vi "read_pressure.vi"(8 "error in (no error)":errorcluster, 10 "Transmitter":string="001", 11 "VISA resource name":refnum<visa-resource-name>) -> (0 "error out":errorcluster, 1 "pressure mbar numeric":dbl format="%_4e", 3 "VISA resource name 2":refnum<visa-resource-name>)   [LabVIEW 2010]
panel:
  out "concatenated string":string
  out "octal integer string":string
  out "sum":u8
  out "unsigned byte array":u8[](array[numeric])
  out "Numeric":u8
  out "read buffer":string
  out "return count":u32
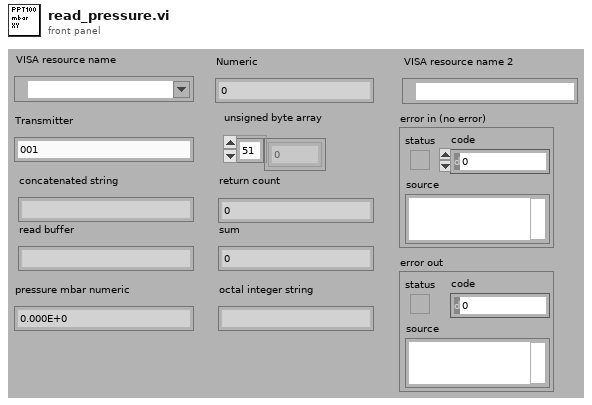
[diagram p1: front panel]
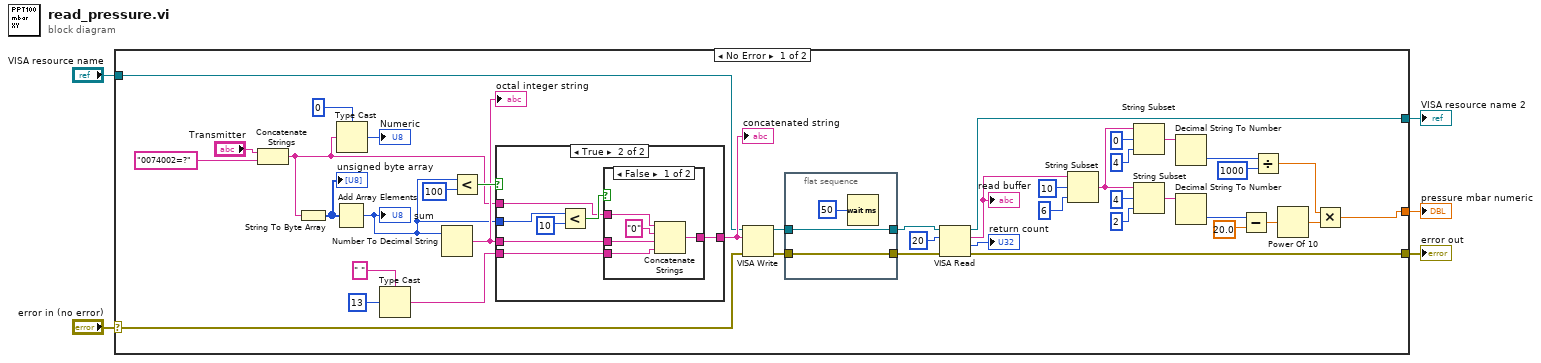
[diagram p0: block diagram]
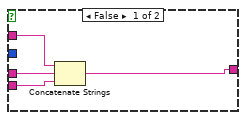
[diagram p2: hidden frame]
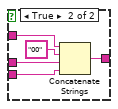
[diagram p3: hidden frame]
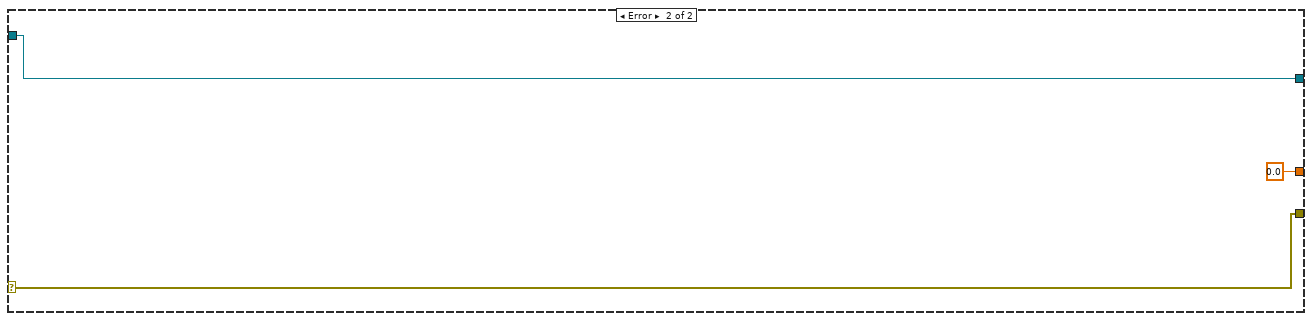
[diagram p4: hidden frame]
diagram:
  n1 = case shown="No Error" "error in (no error)" {
    selector: "error in (no error)" -> [w8 w73]
    tunnel: "VISA resource name" -> [w9 w74]
    tunnel: [w45 w73] -> w4
    tunnel: [w44 w74] -> w2
    tunnel: [w22 0.0] -> w1
    frame No Error {
      n2 = Concatenate Strings("Transmitter", "0074002=?") -> (w10:string)
      n3 = String To Byte Array(string=w10) -> (unsigned byte array=w17:u8[])
      "unsigned byte array" <- w17
      n4 = Add Array Elements(numeric array=w17) -> (sum=w12:u8)
      "sum" <- w12
      n5 = Type Cast(type=u8 0, x=w10) -> (*(type *) &x=→"Numeric":u8)
      n6 = Type Cast(type=" ", x=u8 13 ("Numeric 2")) -> (*(type *) &x=w14:string)
      n7 = Number To Decimal String(number=w12) -> (decimal integer string=w13:string)  [unwired: 1 in]
      "octal integer string" <- w13
      n8 = Less?(x=w12, y=u8 100) -> (x < y?=w15:bool)
      n9 = case shown="True" w15 {
        tunnel: w10 -> [w51 w53]
        tunnel: w14 -> [w49 w55]
        tunnel: w13 -> [w48 w54]
        tunnel: w12 -> [_ w58]
        tunnel: [w50 w52] -> w11
        frame False {
          n10 = Concatenate Strings(w51, w48, w49) -> (w50:string)
        }
        frame True {
          n11 = Less?(x=w58, y=u8 10) -> (x < y?=w56:bool)
          n12 = case shown="False" w56 {
            tunnel: w55 -> [w62 w67]
            tunnel: w54 -> [w61 w66]
            tunnel: w53 -> [w60 w65]
            tunnel: [w59 w64] -> w52
            frame False {
              n13 = Concatenate Strings(w60, "0" ("string"), w61, w62) -> (w59:string)
            }
            frame True {
              n14 = Concatenate Strings(w65, "00" ("string"), w66, w67) -> (w64:string)
            }
          }
        }
      }
      "concatenated string" <- w11
      n15 = VISA Write(VISA resource name=w9, write buffer=w11, error in (no error)=w8) -> (VISA resource name out=w7:refnum<visa-resource-name>, error out=w6:errorcluster)  [unwired: 1 out]
      n16 = flat-sequence {
        tunnel: [w69] -> w41
        tunnel: w6 -> [w70]
        tunnel: [w70] -> w42
        tunnel: w7 -> [w69]
        frame #0 {
          n17 = Wait (ms)(milliseconds to wait=u32 50) -> ()  [unwired: 1 out]
        }
      }
      n18 = VISA Read(VISA resource name=w41, byte count=u32 20, error in (no error)=w42) -> (VISA resource name out=w44:refnum<visa-resource-name>, read buffer=w39:string, return count=→"return count":u32, error out=w45:errorcluster)
      "read buffer" <- w39
      n19 = String Subset(string=w39, offset (0)=10, length (rest)=6 ("length (rest)")) -> (substring=w35:string)
      n20 = String Subset(string=w35, offset (0)=0, length (rest)=4 ("length (rest)")) -> (substring=w31:string)
      n21 = String Subset(string=w35, offset (0)=4, length (rest)=2 ("length (rest)")) -> (substring=w28:string)
      n22 = Decimal String To Number(string=w31) -> (number=w30:i32)  [unwired: 2 in, 1 out]
      n23 = Decimal String To Number(string=w28) -> (number=w26:i32)  [unwired: 2 in, 1 out]
      n24 = Subtract(x=w26, y=20.0) -> (x-y=w24:dbl)
      n25 = Divide(x=w30, y=1000) -> (x/y=w25:dbl)
      n26 = Power Of 10(x=w24) -> (10^x=w23:dbl)
      n27 = Multiply(x=w25, y=w23) -> (x*y=w22:dbl)
    }
    frame Error {
    }
  }
  "error out" <- w4
  "VISA resource name 2" <- w2
  "pressure mbar numeric" <- w1
